vi "testmove.vi"(9 "p_TargetWavelength":dbl, 11 "reference":refnum<k7>) -> (0 "CurrentWavelength":dbl, 1 "MovetoWavelength":i32, 2 "CurrentAngle":dbl, 3 "Device reference out":refnum<k7>, 4 "Timed Out":bool, 5 "Device moved":bool)   [LabVIEW 2019]
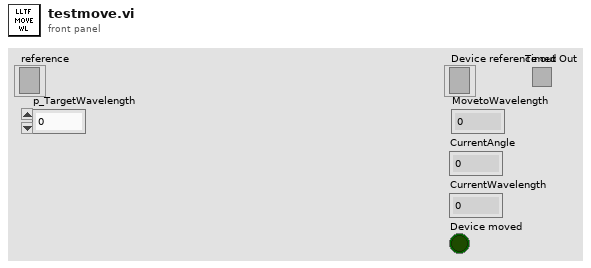
[diagram p1: front panel]
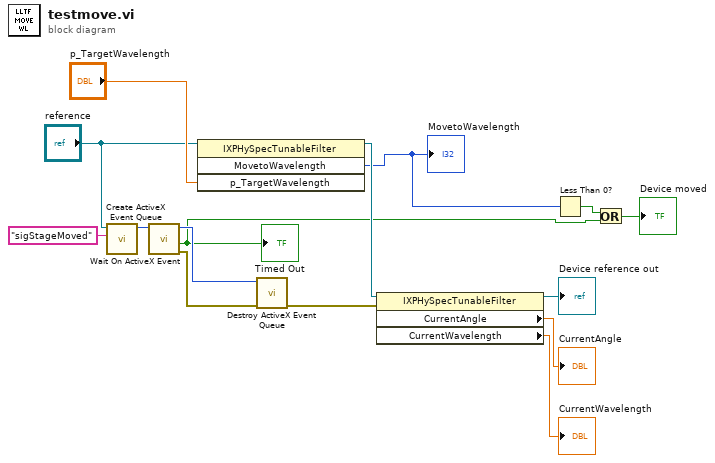
[diagram p0: block diagram]
diagram:
  n1 = call <vilib>:"Create ActiveX Event Queue.vi"("Event Name"="sigStageMoved", "Automation Refnum"="reference") -> ("Event Queue"=w7:i32)  [unwired: 4 in, 1 out]
  n2 = call <vilib>:"Wait On ActiveX Event.vi"("Event Queue"=w7) -> ("error out"=w10:errorcluster, "Timed Out"=w2:bool, "Event Queue Out"=w9:i32)  [unwired: 3 in, 1 out]
  "Timed Out" <- w2
  n3 = invoke class="IXPHySpecTunableFilter" method="MovetoWavelength"(reference="reference", "p_TargetWavelength"="p_TargetWavelength") -> (reference out=w14:refnum<k7>, "MovetoWavelength"=w3:i32)  [unwired: 2 in, 2 out]
  "MovetoWavelength" <- w3
  n4 = call <vilib>:"Destroy ActiveX Event Queue.vi"("error in (no error)"=w10, "Event Queue"=w9) -> ("error out"=w6:errorcluster)  [unwired: 5 in]
  n5 = property class="IXPHySpecTunableFilter"(reference=w14, error in=w6) -> (reference out=→"Device reference out":refnum<k7>, "CurrentAngle"=→"CurrentAngle":dbl, "CurrentWavelength"=→"CurrentWavelength":dbl)  [unwired: 1 out]
  n6 = Less Than 0?(x=w3) -> (x < 0?=w4:bool)
  n7 = Or(x=w4, y=w2) -> (x .or. y?=→"Device moved":bool)
